vi "Error Code and Source Clear.vi"(5 "always (F)":bool, 6 "error in":errorcluster) -> (0 "error out":errorcluster)   [LabVIEW 2020]
doc: "This function clears the error cluster code and source fields when the error status is clear."
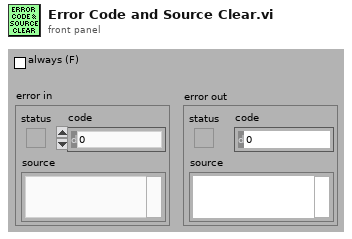
[diagram p1: front panel]
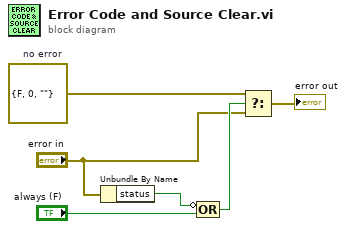
[diagram p0: block diagram]
diagram:
  w1 = errorcluster {"status"=FALSE, "code"=0, "source"=""}  # no error
  n1 = Unbundle By Name("error in") -> ("status"=w3:bool)
  n2 = Compound Arithmetic op=OR(invert w3, "always (F)") -> (w6:bool)
  n3 = Select(t=w1, s=w6, f="error in") -> (s? t:f=→"error out":errorcluster)
